vi "Get Port Status.vi"(8 "error in (no error)":errorcluster, 10 "Port":dbl, 11 "NXP in":refnum<class "NXP.lvclass">) -> (0 "error out":errorcluster, 3 "NXP out":refnum<class "NXP.lvclass">)   [LabVIEW 2020, in "NXP.lvclass"]
doc: "Método heredado del padre con un override"
uses:
  NXP.lvclass
  c5a51af8-9a6b-4b03-996c-9a9038ab4fd5.vi
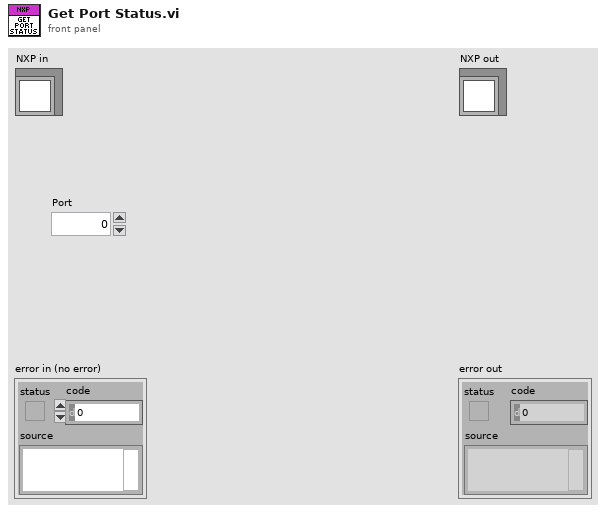
[diagram p1: front panel]
types:
  T1 = typedef "Serial device.lvclass/Brand combobox.ctl" = string
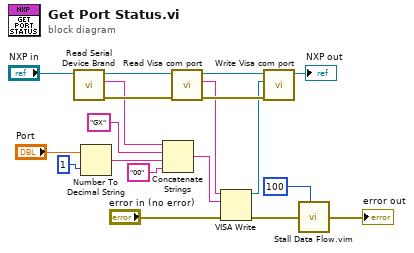
[diagram p0: block diagram]
diagram:
  n1 = call-dynamic "Read Serial Device Brand.vi"("Serial device in"="NXP in") -> ("error out"=w18:errorcluster, "Serial Device Brand"=w8:T1, "Serial device out"=w19:refnum<class "NXP.lvclass">)  [unwired: 8 in]
  n2 = Number To Decimal String(number="Port", width (-)=i16 1) -> (decimal integer string=w13:string)
  n3 = Concatenate Strings(w8, "GX" ("string"), w13, "00" ("string")) -> (w5:string)
  n4 = call-dynamic "Read Visa com port.vi"("error in (no error)"=w18, "Serial device in"=w19) -> ("error out"=w16:errorcluster, "Visa com port"=w4:string, "Serial device out"=w17:refnum<class "NXP.lvclass">)  [unwired: 7 in]
  n5 = VISA Write(VISA resource name=w4, write buffer=w5, error in (no error)="error in (no error)") -> (VISA resource name out=w1:refnum<visa-resource-name>, error out=w7:errorcluster)  [unwired: 1 out]
  n6 = call-dynamic "Write Visa com port.vi"("error in (no error)"=w16, "Visa com port"=w1, "Serial device in"=w17) -> ("Serial device out"=→"NXP out":refnum<class "NXP.lvclass">)  [unwired: 7 in, 1 out]
  n7 = call "Stall Data Flow.vim"("value in"=w7, "milliseconds to wait"=u32 100) -> ("value out"=→"error out":errorcluster)  [unwired: 1 out]
